vi "recycle bin.vi"() -> ()   [LabVIEW 2013]
panel:
  out "Signal 1":dynamicdata(graph)
  out "Signal 4":dynamicdata(graph)
  out "Signal 3":dynamicdata(graph)
  out "Signal 2":dynamicdata(graph)
  in  "address":string
  out "Array 2":dbl[](array[numeric])
  out "Array":dbl[](array[numeric])
  in  "Cluster":T1
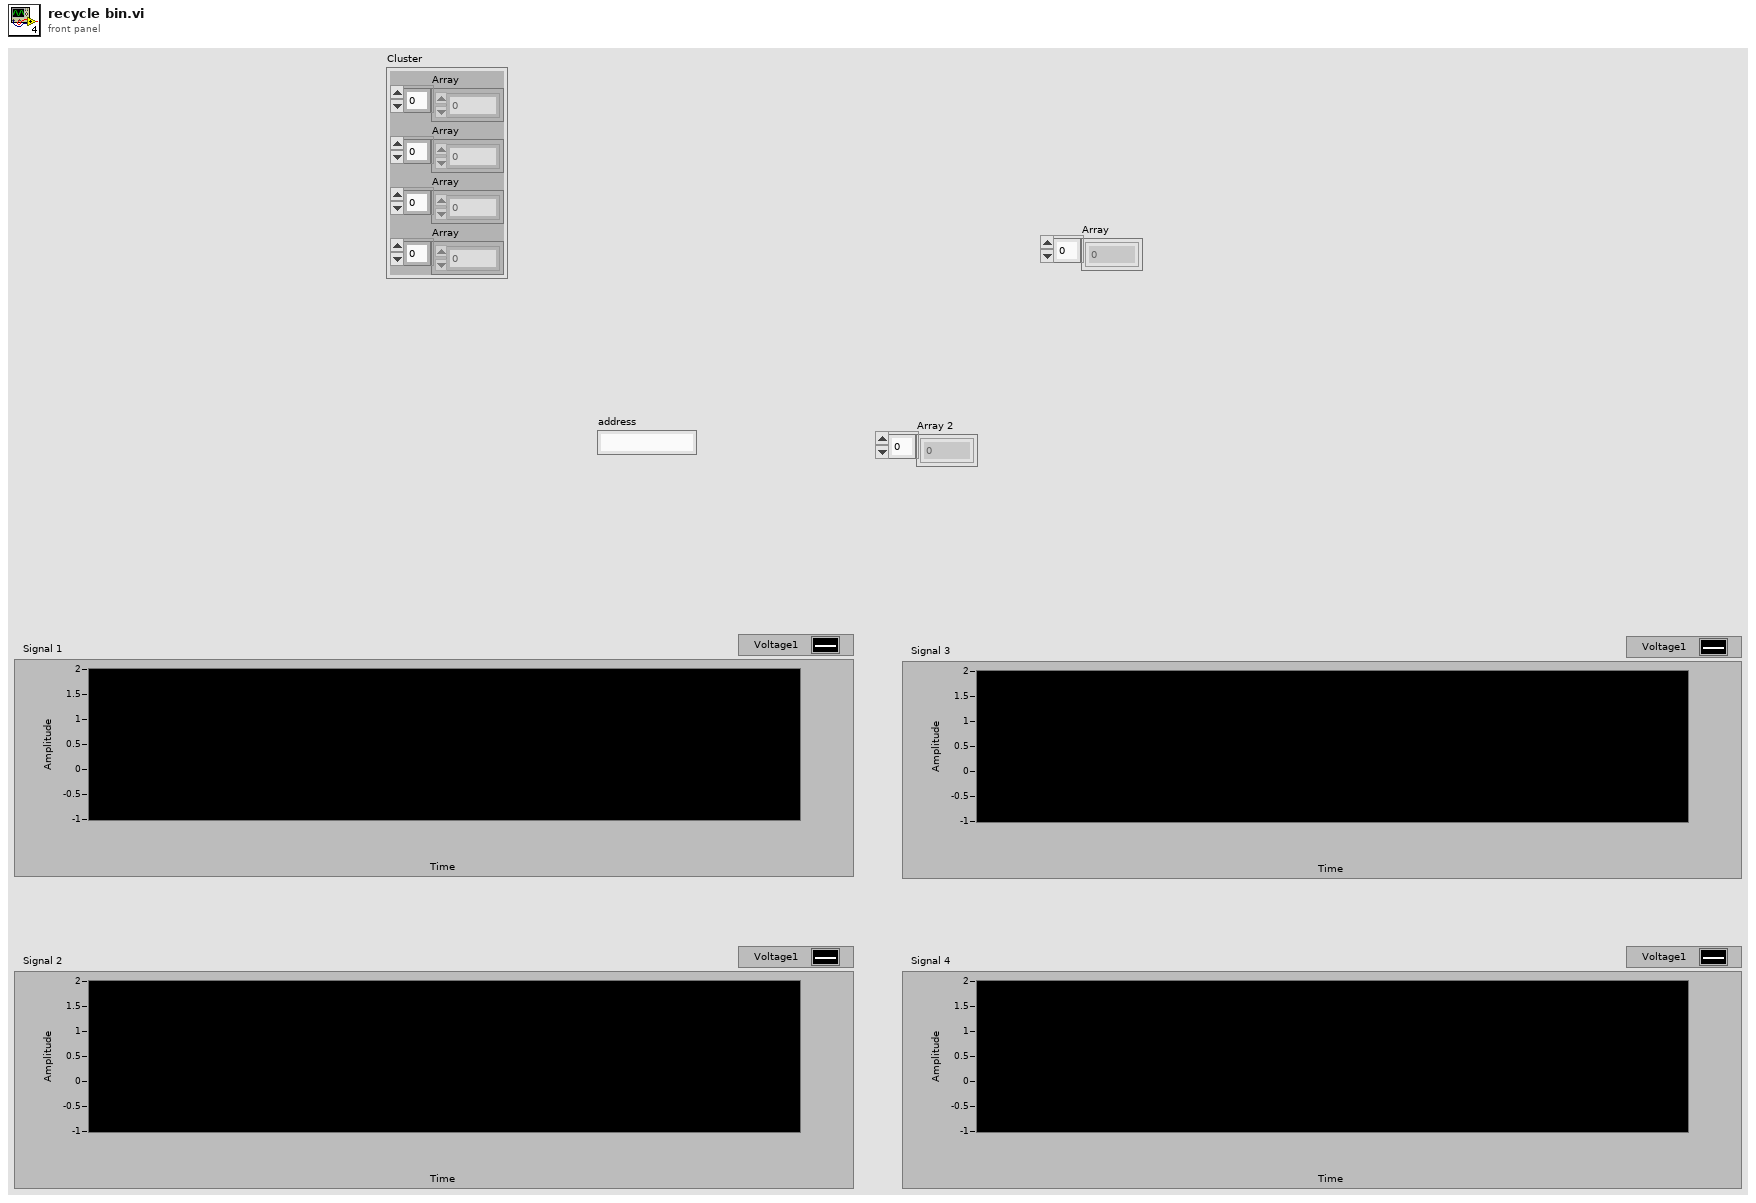
[diagram p1: front panel]
types:
  T1 = cluster{"Array":dbl[], "Array":dbl[], "Array":dbl[], "Array":dbl[]}
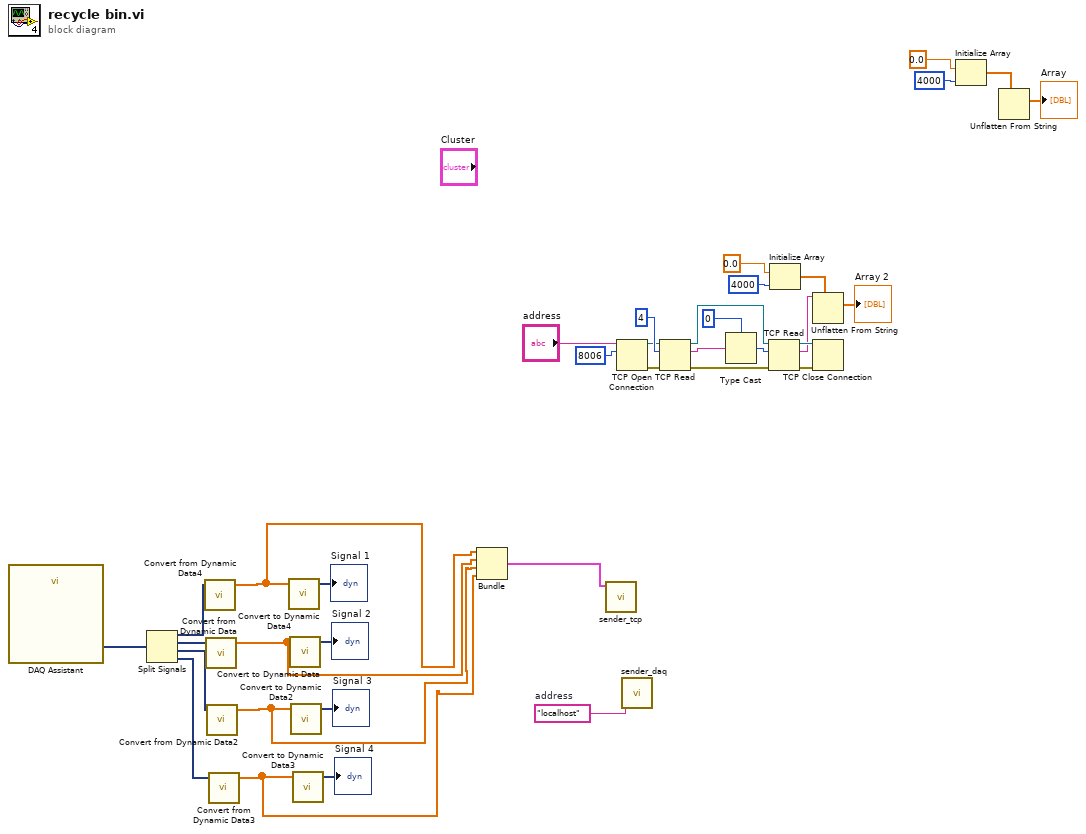
[diagram p0: block diagram]
diagram:
  w12 = "localhost"  # address
  n1 = call "DAQ Assistant"() -> ("data"=w15:dynamicdata)  [unwired: 17 in, 2 out]
  n2 = Split Signals(w15) -> (w8:dynamicdata, w14:dynamicdata, w7:dynamicdata, w6:dynamicdata)  [unwired: 4 in]
  n3 = call "Convert from Dynamic Data4"("Dynamic Data Type"=w8) -> ("Array"=w5:dbl[])  [unwired: 3 in]
  n4 = call "Convert from Dynamic Data"("Dynamic Data Type"=w14) -> ("Array"=w4:dbl[])  [unwired: 3 in]
  n5 = call "Convert from Dynamic Data2"("Dynamic Data Type"=w7) -> ("Array"=w3:dbl[])  [unwired: 3 in]
  n6 = call "Convert from Dynamic Data3"("Dynamic Data Type"=w6) -> ("Array"=w2:dbl[])  [unwired: 3 in]
  n7 = call "Convert to Dynamic Data4"("Array"=w5) -> ("Dynamic Data Type"=→"Signal 1":dynamicdata)  [unwired: 3 in]
  n8 = call "Convert to Dynamic Data"("Array"=w4) -> ("Dynamic Data Type"=→"Signal 2":dynamicdata)  [unwired: 3 in]
  n9 = call "Convert to Dynamic Data2"("Array"=w3) -> ("Dynamic Data Type"=→"Signal 3":dynamicdata)  [unwired: 3 in]
  n10 = call "Convert to Dynamic Data3"("Array"=w2) -> ("Dynamic Data Type"=→"Signal 4":dynamicdata)  [unwired: 3 in]
  n11 = Bundle("Array"=w5, "Array"=w4, "Array"=w3, "Array"=w2) -> (w1:T1)  [unwired: 1 in]
  n12 = call "sender_tcp.vi"("Cluster"=w1) -> ()  [unwired: 11 in]
  n13 = TCP Open Connection(address="address", remote port or service name=8006) -> (connection ID=w21:refnum<k5>, error out=w20:errorcluster)  [unwired: 3 in]
  n14 = call "sender_daq.vi"("address"=w12) -> ()  [unwired: 11 in]
  n15 = TCP Read(connection ID=w21, bytes to read=4, error in (no error)=w20) -> (connection ID out=w24:refnum<k5>, data out=w29:string, error out=w26:errorcluster)  [unwired: 2 in]
  n16 = Type Cast(type=0, x=w29) -> (*(type *) &x=w30:i32)
  n17 = TCP Read(connection ID=w24, bytes to read=w30, error in (no error)=w26) -> (connection ID out=w25:refnum<k5>, data out=w19:string, error out=w27:errorcluster)  [unwired: 2 in]
  n18 = Initialize Array(0.0, 4000) -> (w16:dbl[])
  n19 = Unflatten From String(type=w16, binary string=w19) -> (value=→"Array 2":dbl[])  [unwired: 3 in, 2 out]
  n20 = TCP Close Connection(connection ID=w25, error in (no error)=w27) -> ()  [unwired: 1 in, 2 out]
  n21 = Initialize Array(0.0, 4000) -> (w33:dbl[])
  n22 = Unflatten From String(type=w33) -> (value=→"Array":dbl[])  [unwired: 4 in, 2 out]
